vi "Read Measurement (Spectrum Emission Mask).vi"(0 "VISA resource name":refnum<visa-resource-name>, 5 "Timeout (10000 ms)":i32=10000, 11 "error in (no error)":errorcluster) -> (3 "Measurement Data":dbl[](array[numeric]), 4 "VISA resource name out":refnum<visa-resource-name>, 15 "error out":errorcluster)   [LabVIEW 2022 SP3, in "Agilent N934X Series.lvlib"]
doc: "Reads the measurement result from the spectrum analyzer (Spectrum Emission Mask Measurement) ."
uses:
  <instrlib>/Agilent N934X Series/Agilent N934X Series.lvlib
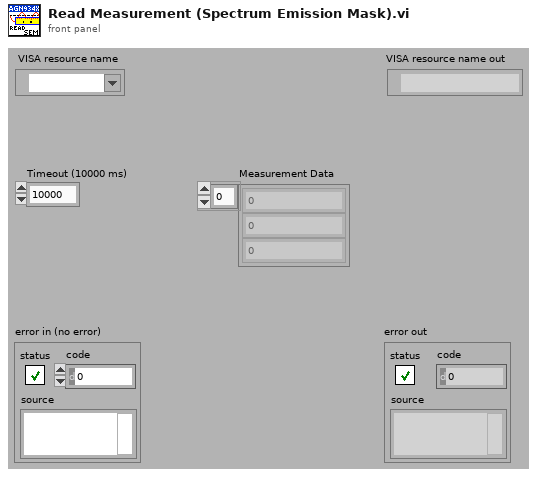
[diagram p1: front panel]
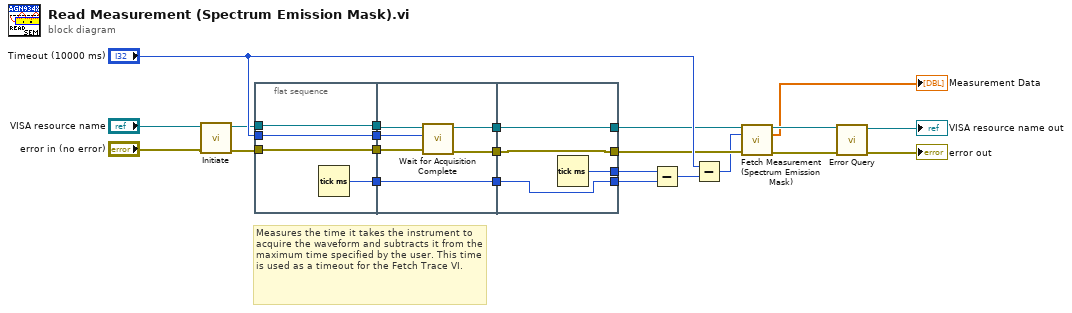
[diagram p0: block diagram]
diagram:
  # "Measures the time it takes the instrument to acquire the waveform and subtracts it from the maximum time specified by the user. This time is used as a timeout for the Fetch Trace VI."
  n1 = call <instrlib>:"Initiate.vi"("error in (no error)"="error in (no error)", "VISA resource name"="VISA resource name") -> ("error out"=w8:errorcluster, "VISA resource name out"=w7:refnum<visa-resource-name>)  [unwired: 8 in]
  n2 = flat-sequence {
    tunnel: [w27] -> w19
    tunnel: w7 -> [w26]
    tunnel: [w26] -> w18
    tunnel: w8 -> [w25]
    tunnel: [w25] -> w17
    tunnel: "Timeout (10000 ms)" -> [w24]
    tunnel: [w24] -> w16
    tunnel: w19 -> [w33]
    tunnel: [w33] -> w15
    tunnel: [w31] -> w14
    tunnel: [w32] -> w13
    tunnel: w18 -> [w30]
    tunnel: w17 -> [w28]
    tunnel: w16 -> [w29]
    tunnel: [w36] -> w21
    tunnel: w15 -> [w36]
    tunnel: [w37] -> w22
    tunnel: [w35] -> w5
    tunnel: w14 -> [w35]
    tunnel: [w34] -> w6
    tunnel: w13 -> [w34]
    frame #0 {
      n3 = Tick Count (ms)() -> (millisecond timer value=w27:u32)
    }
    frame #1 {
      n4 = call <instrlib>:"Wait for Acquisition Complete.vi"("error in (no error)"=w28, "Maximum Time (10000 ms)"=w29, "VISA resource name"=w30) -> ("error out"=w32:errorcluster, "VISA resource name out"=w31:refnum<visa-resource-name>)  [unwired: 7 in]
    }
    frame #2 {
      n5 = Tick Count (ms)() -> (millisecond timer value=w37:u32)
    }
  }
  n6 = Subtract(x=w22, y=w21) -> (x-y=w23:u32)
  n7 = Subtract(x="Timeout (10000 ms)", y=w23) -> (x-y=w4:u32)
  n8 = call <instrlib>:"Fetch Measurement (Spectrum Emission Mask).vi"("VISA resource name"=w5, "Timeout (10000 ms)"=w4, "error in (no error)"=w6) -> ("VISA resource name out"=w2:refnum<visa-resource-name>, "Measurement Data"=→"Measurement Data":dbl[], "error out"=w3:errorcluster)  [unwired: 10 in]
  n9 = call <instrlib>:"Error Query.vi"("error in (no error)"=w3, "VISA resource name"=w2) -> ("error out"=→"error out":errorcluster, "VISA resource name out"=→"VISA resource name out":refnum<visa-resource-name>)  [unwired: 6 in, 2 out]
